vi "Energy and Capacity.vi"(9 "Voltage":dbl=1.5, 10 "Cycle":i32, 11 "Initial Capacity  (mAh) in":dbl=2500.0) -> (0 "Current (mA)":dbl[](array[numeric]), 1 "Voltage (V)":dbl[](array[numeric]), 2 "Energy (Wh)":dbl, 3 "Capacity  (mAh)":dbl, 4 "Pass":bool)   [LabVIEW 2020]
uses:
  SupportVIs/Scalar Polynomial Evaluation (DBL).vi
  SupportVIs/NI_AALPro.lvlib
  SupportVIs/NI_MABase.lvlib
panel:
  out "Waveform Graph":waveform(dbl)[](graph)
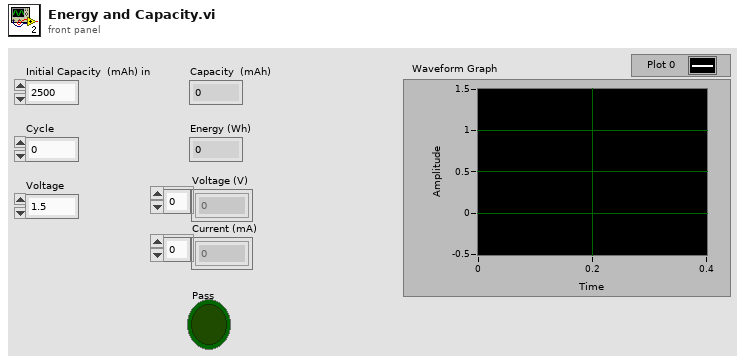
[diagram p1: front panel]
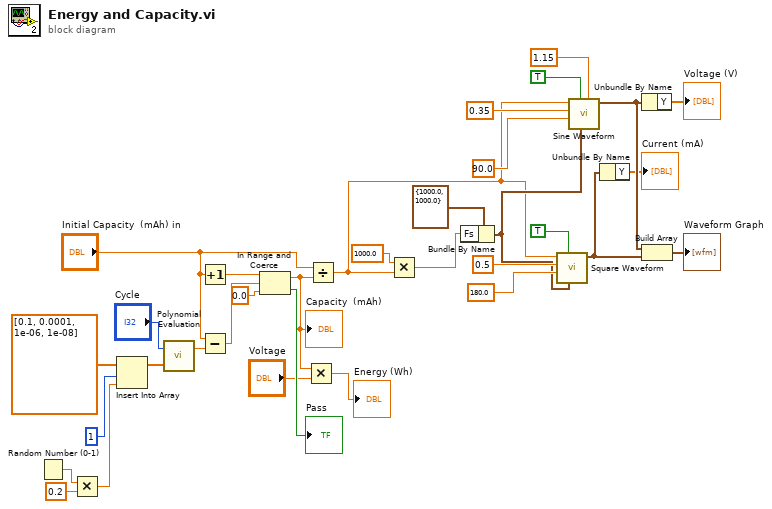
[diagram p0: block diagram]
diagram:
  n1 = Random Number (0-1)() -> (number: 0 to 1=w22:dbl)
  n2 = Multiply(x=w22, y=0.2) -> (x*y=w21:dbl)
  n3 = Insert Into Array(array=dbl[] [0.1, 0.0001, 1e-06, 1e-08] ("P(x)"), index=1, new element=w21) -> (w24:dbl[])
  n4 = call-poly "Polynomial Evaluation.vi"("P(x)"=w24, "a"="Cycle") -> ("P(a)"=w26:dbl)  [unwired: 1 out]
  n5 = Increment(x="Initial Capacity  (mAh) in") -> (x+1=w28:dbl)
  n6 = Subtract(x="Initial Capacity  (mAh) in", y=w26) -> (x-y=w27:dbl)
  n7 = In Range and Coerce(upper limit=w28, x=w27, lower limit=0.0) -> (coerced(x)=w8:dbl, In Range?=→"Pass":bool)
  "Capacity  (mAh)" <- w8
  n8 = Multiply(x=w8, y="Voltage") -> (x*y=→"Energy (Wh)":dbl)
  n9 = Divide(x="Initial Capacity  (mAh) in", y=w8) -> (x/y=w9:dbl)
  n10 = Multiply(x=1000.0, y=w9) -> (x*y=w10:dbl)
  n11 = Bundle By Name(cluster=cluster{"Fs":dbl, "#s":dbl} {"Fs"=1000.0, "#s"=1000.0} ("sampling info"), "Fs"=w10) -> (w12:cluster{"Fs":dbl, "#s":dbl})
  n12 = call "Square Waveform.vi"("sampling info"=w12, "reset signal"=TRUE, "phase"=180.0, "amplitude"=0.5, "frequency"=w9) -> ("signal out"=w5:waveform(dbl))  [unwired: 5 in, 1 out]
  n13 = call "Sine Waveform.vi"("offset"=1.15, "sampling info"=w12, "reset signal"=TRUE, "phase"=90.0, "amplitude"=0.35, "frequency"=w9) -> ("signal out"=w6:waveform(dbl))  [unwired: 4 in, 1 out]
  n14 = Unbundle By Name(w5) -> ("Y"=→"Current (mA)":dbl[])
  n15 = Unbundle By Name(w6) -> ("Y"=→"Voltage (V)":dbl[])
  n16 = Build Array(w6, w5) -> (→"Waveform Graph":waveform(dbl)[])
